vi "LOGIC.vi"() -> ()   [LabVIEW 2020]
panel:
  out "XNOR":bool
  out "XOR logic":bool
  out "NOT logic 2":bool
  out "NAND logic":bool
  out "NOR logic":bool
  in  "Boolean 4":bool
  in  "Boolean":bool
  out "NOT Logic":bool
  out "OR logic":bool
  out "AND logic":bool
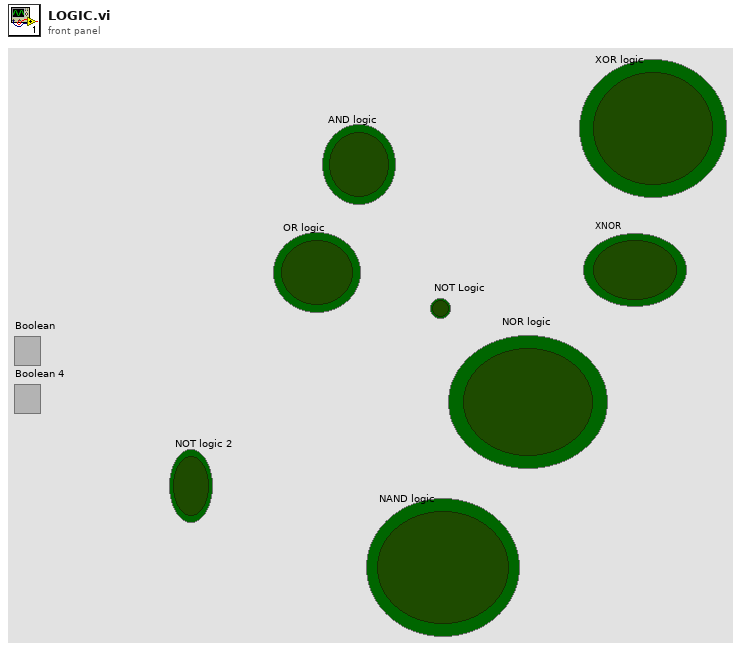
[diagram p1: front panel]
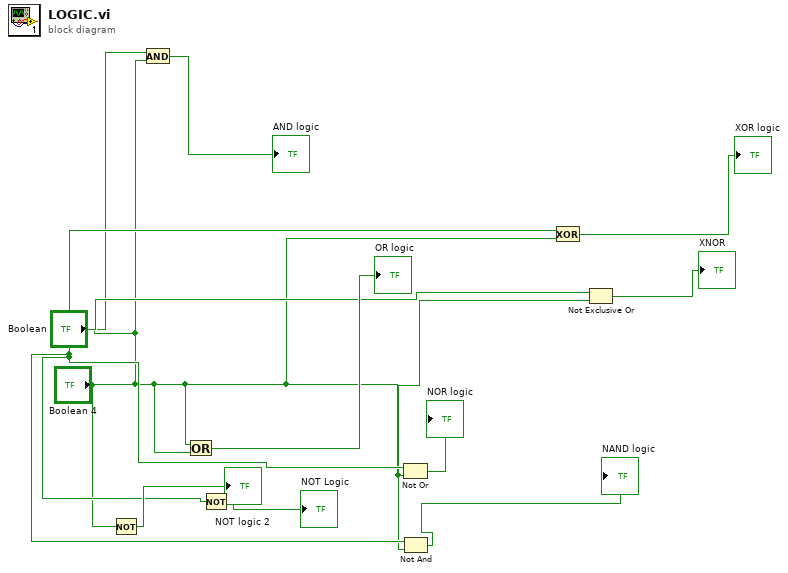
[diagram p0: block diagram]
diagram:
  n1 = Not(x="Boolean 4") -> (.not. x?=→"NOT logic 2":bool)
  n2 = And(x="Boolean 4", y="Boolean 4") -> (x .and. y?=→"AND logic":bool)
  n3 = Or(x="Boolean 4", y="Boolean 4") -> (x .or. y?=→"OR logic":bool)
  n4 = Not(x="Boolean") -> (.not. x?=→"NOT Logic":bool)
  n5 = Not Or(1:"Boolean 4", 2:"Boolean") -> (0:→"NOR logic":bool)
  n6 = Not And(1:"Boolean 4", 2:"Boolean") -> (0:→"NAND logic":bool)
  n7 = Exclusive Or(1:"Boolean 4", 2:"Boolean") -> (0:→"XOR logic":bool)
  n8 = Not Exclusive Or(1:"Boolean 4", 2:"Boolean") -> (0:→"XNOR":bool)
